vi "WriteStrainTCPToTDMS.vi"(0 "TDMS In":refnum<k34>, 1 "Qty of Optical Lines":string, 2 "LineNumber":string, 3 "Peak Powers":string[][](array[string]), 5 "OpticalLineNumber":string[](array[string]), 7 "Time":string, 9 "Qty of FBG's":string[](array[string]), 11 "error in (no error)":errorcluster, 12 "System Status":string[][](array[string]), 13 "Date":string, 14 "Peak Wavelengths":string[][](array[string])) -> (4 "tdms error out":errorcluster)   [LabVIEW 2024]
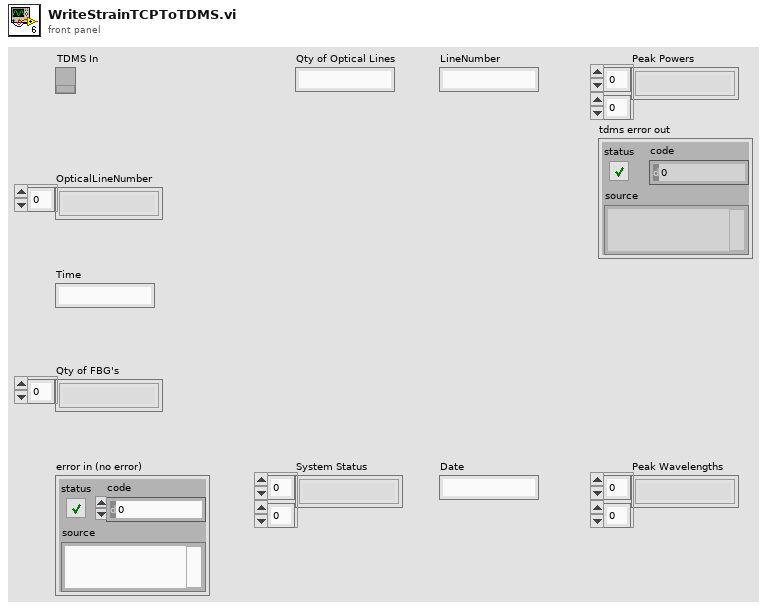
[diagram p1: front panel]
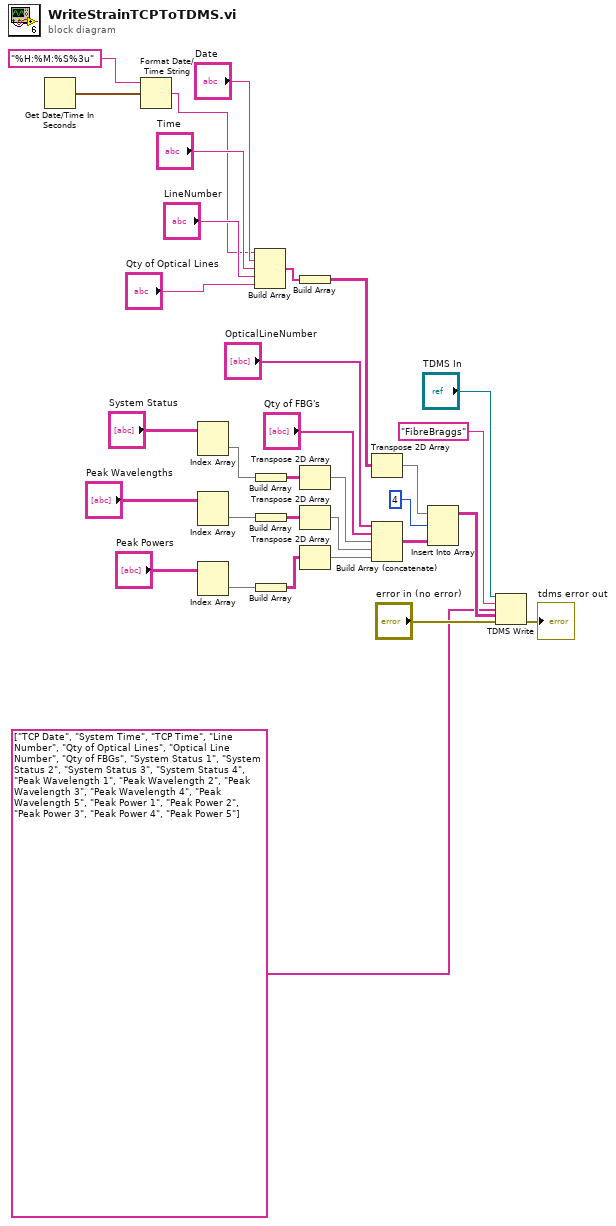
[diagram p0: block diagram]
diagram:
  n1 = Get Date/Time In Seconds() -> (seconds since 1Jan1904=w4:timestamp)
  n2 = Format Date/Time String(time format string (%c)="%H:%M:%S%3u", seconds (now)=w4) -> (date/time string=w2:string)  [unwired: 1 in]
  n3 = Index Array(array="System Status") -> (element=w17:string[])  [unwired: 2 in]
  n4 = Index Array(array="Peak Wavelengths") -> (element=w21:string[])  [unwired: 2 in]
  n5 = Index Array(array="Peak Powers") -> (element=w23:string[])  [unwired: 2 in]
  n6 = Build Array(w2, "Date", "Time", "LineNumber", "Qty of Optical Lines") -> (w26:string[])
  n7 = Build Array(w17) -> (w18:string[][])
  n8 = Build Array(w21) -> (w20:string[][])
  n9 = Build Array(w23) -> (w24:string[][])
  n10 = Build Array(w26) -> (w27:string[][])
  n11 = Transpose 2D Array(2D array=w18) -> (transposed array=w19:string[][])
  n12 = Transpose 2D Array(2D array=w20) -> (transposed array=w22:string[][])
  n13 = Transpose 2D Array(2D array=w24) -> (transposed array=w25:string[][])
  n14 = Transpose 2D Array(2D array=w27) -> (transposed array=w28:string[][])
  n15 = Build Array (concatenate)("OpticalLineNumber", "Qty of FBG's", w19, w22, w25) -> (w29:string[][])
  n16 = Insert Into Array(array=w28, index (row)=4 ("disabled index (col)"), new element=w29) -> (w30:string[][])  [unwired: 1 in]
  n17 = TDMS Write(0:"TDMS In", 5:"FibreBraggs" ("group name in (Untitled)"), 7:string[] ["TCP Date", "System Time", "TCP Time", "Line Number", "Qty of Optical Lines", "Optical Line Number", "Qty of FBGs", "System Status 1", "System Status 2", "System Status 3", "System Status 4", "Peak Wavelength 1", "Peak Wavelength 2", "Peak Wavelength 3", "Peak Wavelength 4", "Peak Wavelength 5", "Peak Power 1", "Peak Power 2", "Peak Power 3", "Peak Power 4", "Peak Power 5"], 9:w30, 11:"error in (no error)") -> (15:→"tdms error out":errorcluster)  [unwired: 1 in, 3 out]
